vi "Actor Core.vi"(8 "error in":errorcluster, 11 "Measure Object in":refnum<class "Resampler.lvclass">) -> (0 "error out":errorcluster, 3 "Actor out":refnum<class "Actor.lvclass">)   [LabVIEW 2024, in "Resampler.lvclass"]
doc: "(<B>Filename</B>: Actor Framework.lvlib:Actor.lvclass:Actor Core.vi)\n\nReceives messages to the actor, reacts to them, and initiates any error handling that may shut the actor down.\n\nDescendant classes may override this VI to append parallel tasks for the actor to complete while it handles messages. Overrides use the Call Parent Method node."
uses:
  Resampler.lvclass
  C:/Nano/fedor2024/labview/LabActor/Template Module/Template Module.lvclass
  C:/Program Files/National Instruments/LabVIEW 2024/vi.lib/ActorFramework/Actor/Actor.lvclass
  <vilib>/ActorFramework/Actor/Actor.lvclass
  Resampler Configuration.ctl
  Template Module/Template Module.lvclass/Template Module.ctl
  <vilib>/ActorFramework/Actor/Actor.lvclass/Actor.ctl
  <vilib>/ActorFramework/Message Enqueuer/Message Enqueuer.lvclass/Message Enqueuer.ctl
  NHMFL_Core/Libraries/Instruments/Results/File Path Result/File Path Result.lvclass
  C:/Nano/fedor2024/labview/NHMFL_Core/Libraries/Instruments/Results/Acquired Result/Acquired Result.lvclass
  Process Object Messages/Process Result Msg/Process Result Msg.lvclass/Process Result Msg.ctl
  Template Module/Read stop event.vi
  <vilib>/ActorFramework/Message Enqueuer/Init from Existing Queue.vi
  <vilib>/ActorFramework/Message Enqueuer/Enqueue.vi
  Process Object Messages/Process Result Msg/Process Result Msg.lvclass
  C:/Program Files/National Instruments/LabVIEW 2024/vi.lib/ActorFramework/Message/Message.lvclass
  <vilib>/ActorFramework/Message Priority Queue/Priority Enqueue.vi
  Process Object/Process Object.lvclass
  <vilib>/ActorFramework/Message Enqueuer/Message Enqueuer.lvclass
  Resampler.lvclass/Resampler.ctl
panel:
  in  "Input file":path
  out "Output file":path
  in  "Re-process":bool
  out "Name":string
  in  "Configuration":T1={"Group"="p", "Reference channel"="", "Channels to resample"=[]}
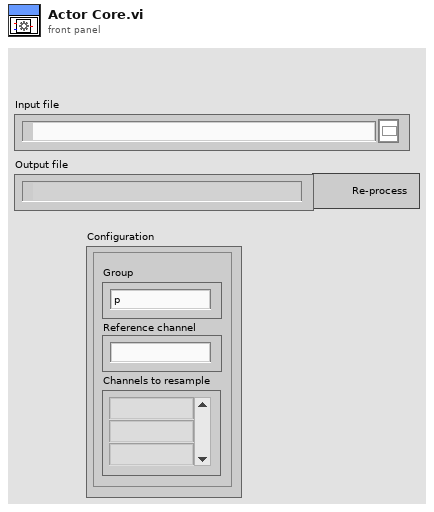
[diagram p1: front panel]
types:
  T1 = typedef "Resampler Configuration.ctl" = cluster{"Group":string, "Reference channel":string, "Channels to resample":string[]}
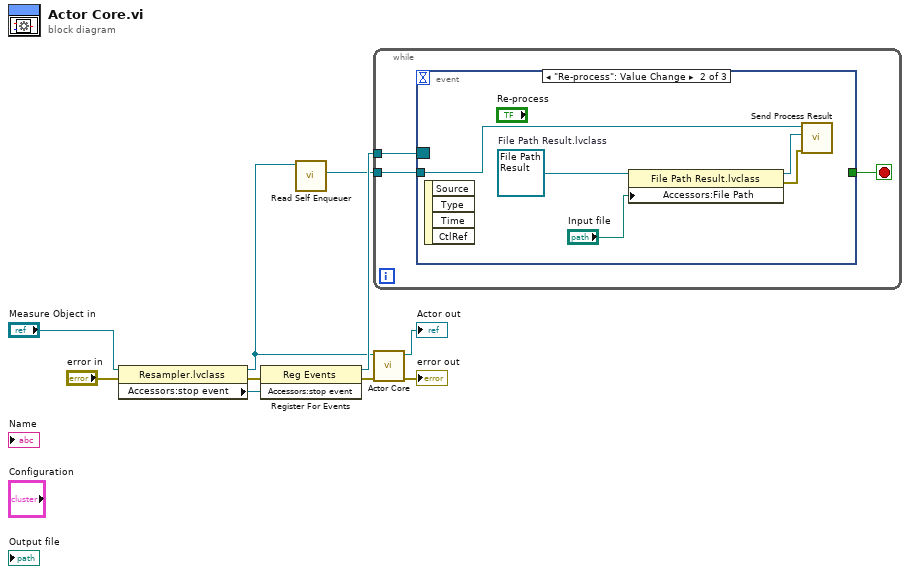
[diagram p0: block diagram]
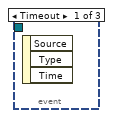
[diagram p2: hidden frame]
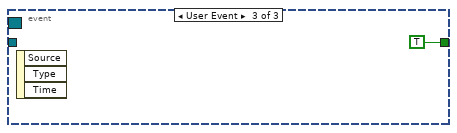
[diagram p3: hidden frame]
diagram:
  n1 = property class="Resampler.lvclass"(reference="Measure Object in", error in="error in") -> (reference out=w3:refnum<class "Resampler.lvclass">, error out=w7:errorcluster, "Accessors:stop event"=w8:refnum<user-event>)
  n2 = register-events(error in=w7, w8) -> (reference out=w6:refnum<event-registration>, error out=w1:errorcluster)  [unwired: 1 in]
  n3 = call <vilib>:"Read Self Enqueuer.vi"("Actor"=w3) -> ("Self Enqueuer"=w5:refnum<class "Message Enqueuer.lvclass">)  [unwired: 10 in]
  n4 = while {
    tunnel: w6 -> [w13]
    tunnel: w5 -> [w11]
    stop <- w12 stop-if-true
    n5 = event shown="[1] \"Re-process\": Value Change" {
      selector: w13 -> [_ _ _]
      dyn-events: _ -> [_ _ _]
      timeout: _ -> [_ _ _]
      tunnel: [_ _ TRUE] -> w12
      tunnel: w11 -> [_ w18 _]
      event Timeout {
        n6 = event-data() -> ()  [unwired: 1 in, 3 out]
      }
      event "Re-process": Value Change {
        w17 = refnum<class "File Path Result.lvclass"> refnum  # File Path Result.lvclass
        n7 = event-data() -> ()  [unwired: 1 in, 4 out]
        n8 = property class="File Path Result.lvclass"(reference=w17, "Accessors:File Path"="Input file") -> (reference out=w16:refnum<class "File Path Result.lvclass">, error out=w15:errorcluster)  [unwired: 1 in]
        n9 = call "Send Process Result.vi"("error in (no error)"=w15, "Result in"=w16, "Message Enqueuer"=w18) -> ()  [unwired: 7 in, 2 out]
      }
      event User Event {
        n10 = event-data() -> ()  [unwired: 1 in, 3 out]
      }
    }
  }
  n11 = call-parent "Actor Core.vi"("error in"=w1, "Measure Object in"=w3) -> ("error out"=→"error out":errorcluster, "Actor out"=→"Actor out":refnum<class "Actor.lvclass">)  [unwired: 8 in]
